vi "Lex {} UnescapedVariable.vi"(8 "Error In":errorcluster) -> (0 "Error Out":errorcluster)   [LabVIEW 2018, in "Tests.lvlib" / "Lexer.lvlib"]
uses:
  Lexer.lvlib
  src/Toolkit/Low-Level/Tokens/UnescapedVariable/UnescapedVariable.lvclass
  <vilib>/addons/_JKI Toolkits/Caraya/classes/Assert/Assert Equal Type_Variant.vi
  src/Toolkit/Low-Level/Tokens/Keyable/Keyable.lvclass
  src/Toolkit/Low-Level/Lexer/Lexer.lvclass
  <vilib>/addons/_JKI Toolkits/Caraya/classes/Test/Test.lvclass
  <vilib>/addons/_JKI Toolkits/Caraya/classes/Assert/Assert.lvclass
  Tests.lvlib
  src/Toolkit/Low-Level/Tokens/Token/Token.lvclass
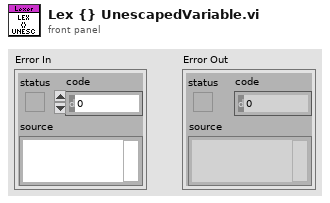
[diagram p1: front panel]
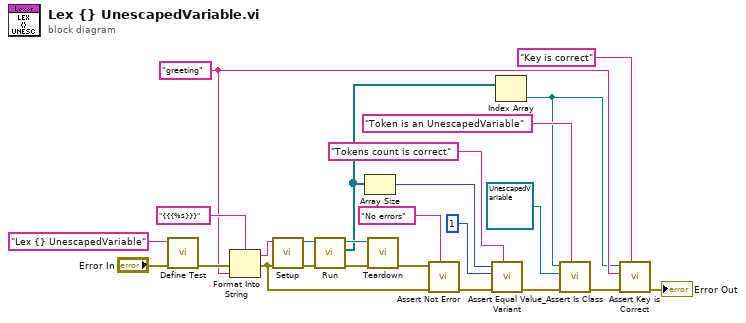
[diagram p0: block diagram]
diagram:
  w12 = "greeting"
  n1 = call <vilib>:"Define Test.vi"("error in (no error)"="Error In", "Label (VI Title)"="Lex {} UnescapedVariable") -> ("error out"=w23:errorcluster)  [unwired: 9 in]
  n2 = Format Into String(format string="{{{%s}}}", error in=w23, w12) -> (resulting string=w1:string, error out=w8:errorcluster)  [unwired: 1 in]
  n3 = call "Setup.vi"("Error In"=w8, "String"=w1) -> ("Error Out"=w6:errorcluster, "Lexer"=w7:refnum<class "Lexer.lvclass">)  [unwired: 8 in]
  n4 = call-dynamic "Run.vi"("Error In"=w6, "Lexer In"=w7) -> ("Error Out"=w4:errorcluster, "Tokens"=w2:refnum<class "Token.lvclass">[], "Lexer Out"=w5:refnum<class "Lexer.lvclass">)  [unwired: 7 in]
  n5 = Array Size(array=w2) -> (size(s)=w19:i32)
  n6 = call "Teardown.vi"("Error In"=w4, "Lexer"=w5) -> ("Error Out"=w3:errorcluster)  [unwired: 9 in]
  n7 = call <vilib>:"Assert Not Error.vi"("Label"="No errors", "error in (no error)"=w8, "Not Error?"=w3) -> ("error out"=w21:errorcluster)  [unwired: 8 in]
  n8 = call <vilib>:"Assert Equal Value_Variant.vi"("Label"="Tokens count is correct", "error in (no error)"=w21, "Y"=1 ("size(s)"), "X"=w19) -> ("error out"=w17:errorcluster)  [unwired: 7 in]
  n9 = Index Array(array=w2) -> (element=w11:refnum<class "Token.lvclass">)  [unwired: 1 in]
  n10 = call "Assert Is Class.vi"("Label"="Token is an UnescapedVariable", "Error In"=w17, "Expected"=refnum<class "UnescapedVariable.lvclass"> refnum ("Mustache.lvlib:Tokens.lvlib:UnescapedVariable.lvclass"), "Actual"=w11) -> ("Error Out"=w10:errorcluster)  [unwired: 7 in]
  n11 = call "Assert Key is Correct.vi"("Label"="Key is correct", "Error In"=w10, "Expected"=w12, "Token"=w11) -> ("Error Out"=→"Error Out":errorcluster)  [unwired: 7 in]
